vi "pipx40 Initialize.vi"(3 "error in (no error)":errorcluster, 4 "reset device":bool=TRUE, 5 "id query":bool=TRUE, 6 "resource name":string="PXI2::15::INSTR") -> (0 "error out":errorcluster, 1 "status":i32 format="%.0x", 2 "instrument handle out":refnum<visa-resource-name>)   [LabVIEW 2011]
doc: "Initializes the card having the specified VISA resource name, claiming whatever system resources it requires.\n\nThe card is initialized in the following ways:\n - the card is opened\n - all output channels are cleared\n - all output channels are unmasked"
uses:
  pipx40_32.dll
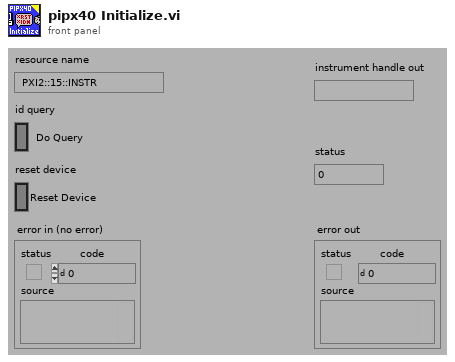
[diagram p1: front panel]
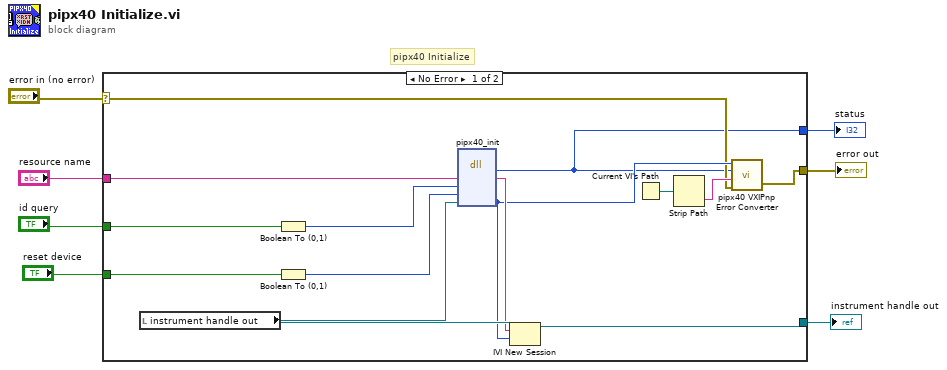
[diagram p0: block diagram]
diagram:
  # "pipx40 Initialize"
  n1 = case shown="No Error" "error in (no error)" {
    selector: "error in (no error)" -> [w12 w22]
    tunnel: [w14 w22] -> w7
    tunnel: [w13 _] -> w6
    tunnel: [w8 _] -> w5
    tunnel: "resource name" -> [w11 _]
    tunnel: "reset device" -> [w10 _]
    tunnel: "id query" -> [w9 _]
    frame No Error {
      n2 = local read "instrument handle out"() -> (w19:refnum<visa-resource-name>)
      n3 = Boolean To (0,1)(Boolean=w9) -> (0, 1=w21:i16)
      n4 = Boolean To (0,1)(Boolean=w10) -> (0, 1=w20:i16)
      n5 = dll-call lib="pipx40_32.dll" fn="pipx40_init" label="pipx40 Initialize"("resource name"=w11, "id query"=w21, "reset device"=w20, "instrument handle"=w19) -> ("status"=w8:i32, "resource name"=w18:string, "instrument handle"=w17:u32)  [unwired: 5 in, 2 out]
      n6 = IVI New Session(9:w17, 10:w18, 11:w19) -> (3:w13:refnum<visa-resource-name>)
      n7 = Current VI's Path() -> (path=w16:path)
      n8 = Strip Path(path=w16) -> (name=w15:string)  [unwired: 1 out]
      n9 = call "pipx40 VXIPnp Error Converter.vi"("error in (no error)"=w12, "name of VI (\"\")"=w15, "VXIPnp error code (0)"=w8, "instrument handle"=w17) -> ("error out"=w14:errorcluster)  [unwired: 1 out]
    }
    frame Error {
    }
  }
  "error out" <- w7
  "instrument handle out" <- w6
  "status" <- w5
